vi "Create Certificate Data Bundles.vi"(0 "Tolerancing Bundle":T1(array[cluster]), 7 "CalChannelsAsFound":string[][](array[string]), 11 "CalChannelsVerify":string[][](array[string])) -> (4 "Data":T2(array[cluster]))   [LabVIEW 2013]
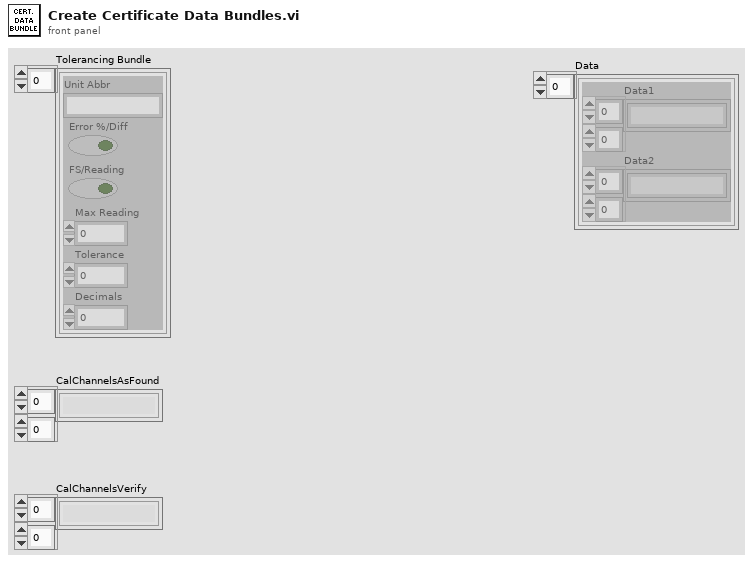
[diagram p1: front panel]
types:
  T1 = cluster{"Unit Abbr":string, "Error %/Diff":bool, "FS/Reading":bool, "Max Reading":dbl, "Tolerance":dbl, "Decimals":i16}[]
  T2 = cluster{"Data1":string[][], "Data2":string[][]}[]
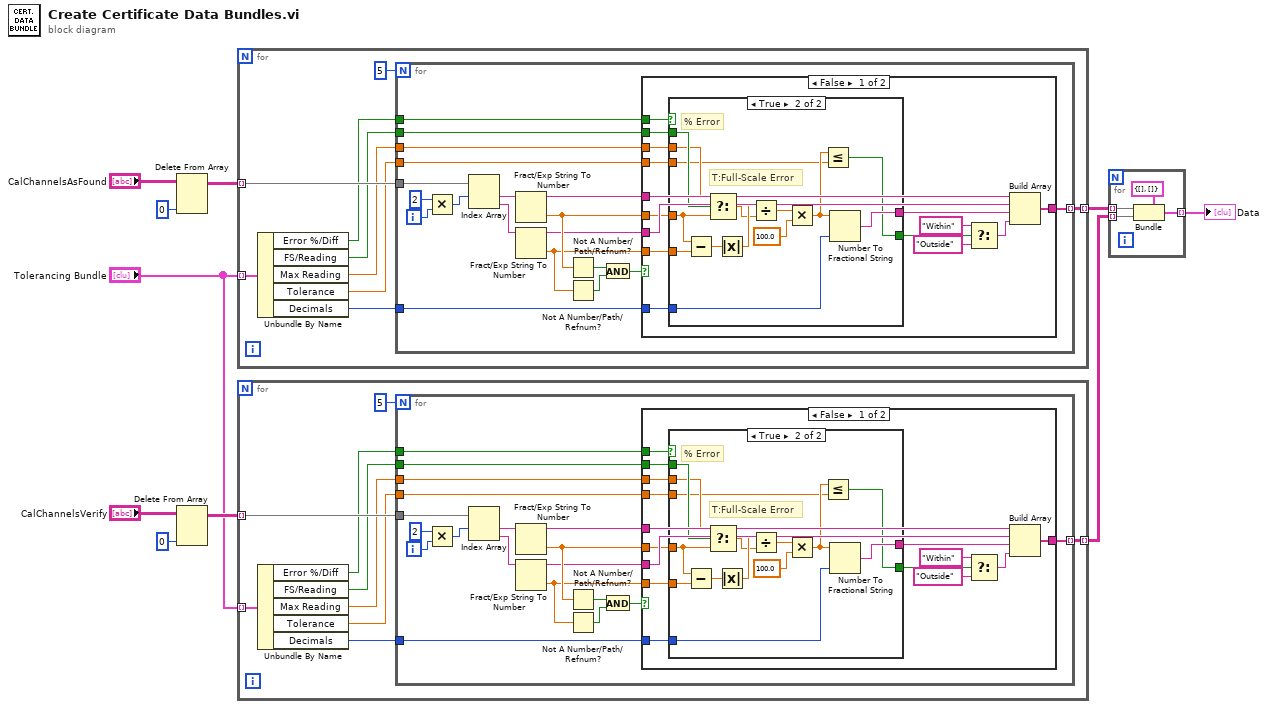
[diagram p0: block diagram]
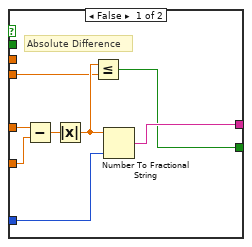
[diagram p2: hidden frame]
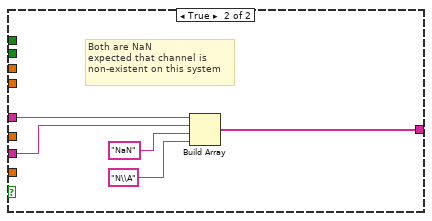
[diagram p3: hidden frame]
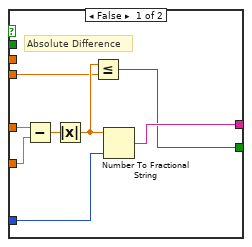
[diagram p4: hidden frame]
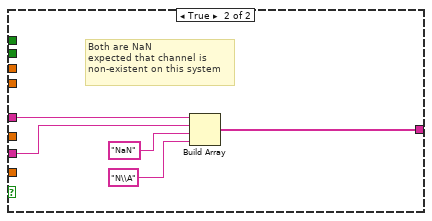
[diagram p5: hidden frame]
diagram:
  n1 = Delete From Array(array="CalChannelsAsFound", index (col)=0 ("disabled index (col)")) -> (array with subset deleted=w8:string[][])  [unwired: 2 in, 1 out]
  n2 = Delete From Array(array="CalChannelsVerify", index (col)=0 ("disabled index (col)")) -> (array with subset deleted=w3:string[][])  [unwired: 2 in, 1 out]
  n3 = for {
    tunnel: w8 -> [w19] mode=indexing
    tunnel: [w17] -> w5 mode=indexing
    tunnel: "Tolerancing Bundle" -> [w16] mode=indexing
    n4 = Unbundle By Name(w16) -> ("Error %/Diff"=w15:bool, "FS/Reading"=w14:bool, "Max Reading"=w13:dbl, "Tolerance"=w12:dbl, "Decimals"=w11:i16)
    n5 = for {
      N: 5 -> [_]
      tunnel: w19 -> [w35]
      tunnel: [w26] -> w17 mode=indexing
      tunnel: w15 -> [w25]
      tunnel: w14 -> [w24]
      tunnel: w13 -> [w23]
      tunnel: w12 -> [w22]
      tunnel: w11 -> [w20]
      i -> [w21]
      n6 = Multiply(x=2, y=w21) -> (x*y=w34:i32)
      n7 = Index Array(array=w35, index #1=w34) -> (element #1=w30:string, element #2=w28:string)  [unwired: 1 in]
      n8 = Fract/Exp String To Number(string=w30) -> (number=w29:dbl)  [unwired: 3 in, 1 out]
      n9 = Fract/Exp String To Number(string=w28) -> (number=w27:dbl)  [unwired: 3 in, 1 out]
      n10 = Not A Number/Path/Refnum?(number/path/refnum=w29) -> (NaN/Path/Refnum?=w33:bool)
      n11 = Not A Number/Path/Refnum?(number/path/refnum=w27) -> (NaN/Path/Refnum?=w32:bool)
      n12 = And(x=w33, y=w32) -> (x .and. y?=w31:bool)
      n13 = case shown="False" w31 {
        tunnel: w30 -> [w50 w78]
        tunnel: w29 -> [w46 _]
        tunnel: w28 -> [w49 w77]
        tunnel: w27 -> [w45 _]
        tunnel: [w51 w74] -> w26
        tunnel: w25 -> [w47 _]
        tunnel: w24 -> [w48 _]
        tunnel: w23 -> [w42 _]
        tunnel: w22 -> [w43 _]
        tunnel: w20 -> [w37 _]
        frame False {
          n14 = case shown="True" w47 {
            tunnel: w48 -> [_ w67]
            tunnel: w46 -> [w59 w65]
            tunnel: w45 -> [w58 w73]
            tunnel: [w56 w68] -> w44
            tunnel: w43 -> [w54 w62]
            tunnel: w42 -> [_ w66]
            tunnel: [w53 w61] -> w38
            tunnel: w37 -> [w52 w60]
            frame False {
              # "Absolute Difference"
              n15 = Subtract(x=w59, y=w58) -> (x-y=w57:dbl)
              n16 = Absolute Value(x=w57) -> (abs(x)=w55:dbl)
              n17 = Less Or Equal?(x=w55, y=w54) -> (x <= y?=w53:bool)
              n18 = Number To Fractional String(number=w55, precision (6)=w52) -> (F-format string=w56:string)  [unwired: 2 in]
            }
            frame True {
              # "T:Full-Scale Error"
              # "% Error"
              n19 = Subtract(x=w65, y=w73) -> (x-y=w72:dbl)
              n20 = Select(t=w66, s=w67, f=w65) -> (s? t:f=w64:dbl)
              n21 = Absolute Value(x=w72) -> (abs(x)=w71:dbl)
              n22 = Divide(x=w71, y=w64) -> (x/y=w70:dbl)
              n23 = Multiply(x=w70, y=100.0) -> (x*y=w63:dbl)
              n24 = Less Or Equal?(x=w63, y=w62) -> (x <= y?=w61:bool)
              n25 = Number To Fractional String(number=w63, precision (6)=w60) -> (F-format string=w68:string)  [unwired: 2 in]
            }
          }
          n26 = Select(t="Within", s=w38, f="Outside") -> (s? t:f=w39:string)
          n27 = Build Array(w50, w49, w44, w39) -> (w51:string[])
        }
        frame True {
          # "Both are NaN\nexpected that channel is\nnon-existent on this system"
          n28 = Build Array(w78, w77, "NaN", "N\\A") -> (w74:string[])
        }
      }
    }
  }
  n29 = for {
    tunnel: w3 -> [w87] mode=indexing
    tunnel: [w85] -> w2 mode=indexing
    tunnel: "Tolerancing Bundle" -> [w84] mode=indexing
    n30 = Unbundle By Name(w84) -> ("Error %/Diff"=w83:bool, "FS/Reading"=w82:bool, "Max Reading"=w81:dbl, "Tolerance"=w80:dbl, "Decimals"=w79:i16)
    n31 = for {
      N: 5 -> [_]
      tunnel: w87 -> [w103]
      tunnel: [w94] -> w85 mode=indexing
      tunnel: w83 -> [w93]
      tunnel: w82 -> [w92]
      tunnel: w81 -> [w91]
      tunnel: w80 -> [w90]
      tunnel: w79 -> [w88]
      i -> [w89]
      n32 = Multiply(x=2, y=w89) -> (x*y=w102:i32)
      n33 = Index Array(array=w103, index #1=w102) -> (element #1=w98:string, element #2=w96:string)  [unwired: 1 in]
      n34 = Fract/Exp String To Number(string=w98) -> (number=w97:dbl)  [unwired: 3 in, 1 out]
      n35 = Fract/Exp String To Number(string=w96) -> (number=w95:dbl)  [unwired: 3 in, 1 out]
      n36 = Not A Number/Path/Refnum?(number/path/refnum=w97) -> (NaN/Path/Refnum?=w101:bool)
      n37 = Not A Number/Path/Refnum?(number/path/refnum=w95) -> (NaN/Path/Refnum?=w100:bool)
      n38 = And(x=w101, y=w100) -> (x .and. y?=w99:bool)
      n39 = case shown="False" w99 {
        tunnel: w98 -> [w118 w146]
        tunnel: w97 -> [w114 _]
        tunnel: w96 -> [w117 w145]
        tunnel: w95 -> [w113 _]
        tunnel: [w119 w142] -> w94
        tunnel: w93 -> [w115 _]
        tunnel: w92 -> [w116 _]
        tunnel: w91 -> [w110 _]
        tunnel: w90 -> [w111 _]
        tunnel: w88 -> [w105 _]
        frame False {
          n40 = case shown="True" w115 {
            tunnel: w116 -> [_ w135]
            tunnel: w114 -> [w127 w133]
            tunnel: w113 -> [w126 w141]
            tunnel: [w124 w136] -> w112
            tunnel: w111 -> [w122 w130]
            tunnel: w110 -> [_ w134]
            tunnel: [w121 w129] -> w106
            tunnel: w105 -> [w120 w128]
            frame False {
              # "Absolute Difference"
              n41 = Subtract(x=w127, y=w126) -> (x-y=w125:dbl)
              n42 = Absolute Value(x=w125) -> (abs(x)=w123:dbl)
              n43 = Less Or Equal?(x=w123, y=w122) -> (x <= y?=w121:bool)
              n44 = Number To Fractional String(number=w123, precision (6)=w120) -> (F-format string=w124:string)  [unwired: 2 in]
            }
            frame True {
              # "T:Full-Scale Error"
              # "% Error"
              n45 = Subtract(x=w133, y=w141) -> (x-y=w140:dbl)
              n46 = Select(t=w134, s=w135, f=w133) -> (s? t:f=w132:dbl)
              n47 = Absolute Value(x=w140) -> (abs(x)=w139:dbl)
              n48 = Divide(x=w139, y=w132) -> (x/y=w138:dbl)
              n49 = Multiply(x=w138, y=100.0) -> (x*y=w131:dbl)
              n50 = Less Or Equal?(x=w131, y=w130) -> (x <= y?=w129:bool)
              n51 = Number To Fractional String(number=w131, precision (6)=w128) -> (F-format string=w136:string)  [unwired: 2 in]
            }
          }
          n52 = Select(t="Within", s=w106, f="Outside") -> (s? t:f=w107:string)
          n53 = Build Array(w118, w117, w112, w107) -> (w119:string[])
        }
        frame True {
          # "Both are NaN\nexpected that channel is\nnon-existent on this system"
          n54 = Build Array(w146, w145, "NaN", "N\\A") -> (w142:string[])
        }
      }
    }
  }
  n55 = for {
    tunnel: w5 -> [w149] mode=indexing
    tunnel: w2 -> [w148] mode=indexing
    tunnel: [w147] -> w4 mode=indexing
    n56 = Bundle(cluster=cluster{"Data1":string[][], "Data2":string[][]} {"Data1"=[], "Data2"=[]}, "Data1"=w149, "Data2"=w148) -> (w147:cluster{"Data1":string[][], "Data2":string[][]})
  }
  "Data" <- w4
